vi "FloatApprox.vi"(2 "y":dbl, 3 "x":dbl) -> (0 "x ~ y?":bool)   [LabVIEW 2016, in "Instrument.Lockin.lvclass"]
doc: "Use to compare floating point numbers. This will check if two numbers are the same to 6 decimal places. Edit block diagram to change tolerance."
uses:
  Instrument.Lockin.lvclass
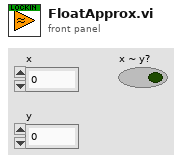
[diagram p1: front panel]
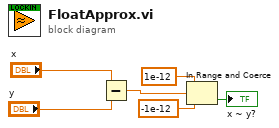
[diagram p0: block diagram]
diagram:
  n1 = Subtract(x="x", y="y") -> (x-y=w3:dbl)
  n2 = In Range and Coerce(upper limit=1e-12, x=w3, lower limit=-1e-12 ("upper limit")) -> (In Range?=→"x ~ y?":bool)  [unwired: 1 out]
